vi "op-init.vi"(0 "Chain IN":bool) -> (4 "Chain OUT":bool)   [LabVIEW 2010, in "LASA Beta.lvrbt"]
uses:
  LASA Beta.lvrbt
  <vilib>/NXT/NXTIO Xnodes/AddressXNode/NXTIOAddress.xnode
  <vilib>/NXT/Subs/MotorXNode.DC Motor Type.ctl
  <vilib>/NXT/Subs/MotorXNode.1DCMotor.ctl
  <vilib>/NXT/Subs/MotorXNode.2DCMotor.ctl
  <vilib>/NXT/Subs/LVHSConnector.ctl
  <vilib>/NXT/NXTIO Xnodes/NXTIOXNode/NXTIO.xnode
  <vilib>/NXT/NXTIO Xnodes/NXTIONodeSubVIs/TETRIX IO Reset Encoders.vi
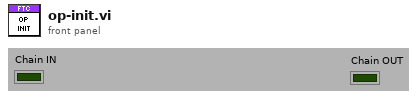
[diagram p1: front panel]
types:
  T1 = typedef "MotorXNode.DC Motor Type.ctl" = enum16{"DC Motor"}
  T2 = cluster{"DC Motor":T1, "Address":i16, "Address":i16}
  T3 = typedef "LVHSConnector.ctl" = cluster{"Hardware":string, "Flattened String":string}
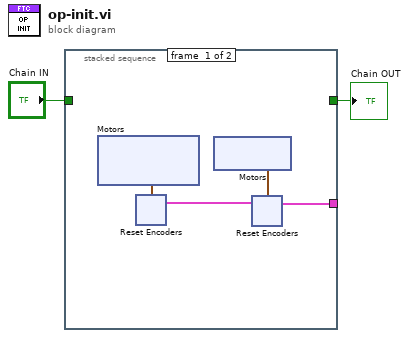
[diagram p0: block diagram]
diagram:
  n1 = stacked-sequence {
    tunnel: "Chain IN" -> [_ w20]
    tunnel: [w3 _] -> _
    tunnel: [_ w20] -> w1
    frame #0 {
      n2 = xnode "Motors"() -> ("DC Motor"=w6:T2)
      n3 = xnode "Reset Encoders"("Motors"=w6) -> ("NXT"=w4:T3)  [unwired: 1 in]
      n4 = xnode "Motors"() -> ("DC Motor"=w5:cluster{"DC Motor":T1, "Address":i16})
      n5 = xnode "Reset Encoders"("Motors"=w5, "NXT"=w4) -> ("NXT"=w3:T3)
    }
    frame #1 {
    }
  }
  "Chain OUT" <- w1
